vi "getConfiguration.vi"(8 "error in (no error)":errorcluster, 11 "Camera in":refnum<class "Camera.lvclass">) -> (0 "error out":errorcluster, 2 "configuration":T2={"exposure_time_s"=nan, "delay_time_s"=nan, "roi"={"x0"=18446744073709551615, "y0"=18446744073709551615, "x1"=18446744073709551615, "y1"=18446744073709551615}, "timestamp_mode"=65535, "pixelrate"=4294967295, "trigger_mode"=65535, "acquire_mode"=65535, "metadata_mode"=65535, "noisefilter_mode"=65535, "binning"={"vert"=65535, "horz"=65535}} {"noisefilter_mode" items=["Undefined"=65535, "OFF"=0, "ON"=1]; "exposure_time_s" format="%#_6f"; "timestamp_mode" items=["Undefined"=65535, "OFF"=0, "Binary"=1, "Binary+ASCII"=2, "ASCII"=3]; "acquire_mode" items=["Undefined"=65535, "auto"=0, "external"=1, "external modulate"=2]; "trigger_mode" items=["Undefined"=65535, "auto sequence"=0, "software trigger"=1, "external exposure start & software trigger"=2, "external exposure control"=3, "external synchronized"=4, "fast external exposure control"=5, "external CDS control"=6, "slow external exposure control"=7, "external synchronized HDSDI"=258]; "metadata_mode" items=["Undefined"=65535, "OFF"=0, "ON"=1]}, 3 "Camera out":refnum<class "Camera.lvclass">)   [LabVIEW 2019, in "Camera.lvclass"]
doc: "Gets the current configuration from the camera."
uses:
  Camera.lvclass
  pco.sdk/TimingControl/TimingControl.lvlib
  pco.sdk/ImageSensor/ImageSensor.lvlib
  pco.sdk/RecordingControl/RecordingControl.lvlib
  Controls/binning.ctl
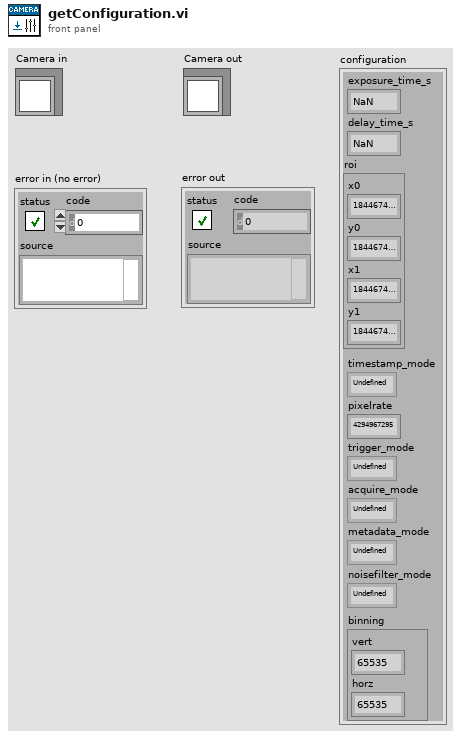
[diagram p1: front panel]
types:
  T1 = typedef "Camera.lvclass/binning.ctl" = cluster{"vert":u16, "horz":u16}
  T2 = cluster{"exposure_time_s":dbl, "delay_time_s":dbl, "roi":cluster{"x0":u64, "y0":u64, "x1":u64, "y1":u64}, "timestamp_mode":u16, "pixelrate":u32, "trigger_mode":u16, "acquire_mode":u16, "metadata_mode":u16, "noisefilter_mode":u16, "binning":T1}
  T3 = cluster{"exposure_time_s":dbl, "delay_time_s":dbl, "roi":cluster{"x0":u64, "y0":u64, "x1":u64, "y1":u64}, "timestamp_mode":u16, "pixelrate":u32, "trigger_mode":u16, "acquire_mode":u16, "metadata_mode":u16, "noisefilter_mode":u16, "binning":cluster{"vert":u16, "horz":u16}}
  T4 = cluster{"wSensorTypeDESC":u16, "wSensorSubTypeDESC":u16, "wMaxHorzResStdDESC":u16, "wMaxVertResStdDESC":u16, "wMaxHorzResExtDESC":u16, "wMaxVertResExtDESC":u16, "wDynResDESC":u16, "wMaxBinHorzDESC":u16, "wBinHorzSteppingDESC":u16, "wMaxBinVertDESC":u16, "wBinVertSteppingDESC":u16, "wRoiHorStepsDESC":u16, "wRoiVertStepsDESC":u16, "wNumADCsDESC":u16, "wMinSizeHorzDESC":u16, "dwPixelRateDESC":u32[], "wConvFactDESC":u16[], "sCoolingSetpoints":i16[], "wSoftRoiHorStepsDESC":u16, "wSoftRoiVertStepsDESC":u16, "wIRDESC":u16, "wMinSizeVertDESC":u16, "dwMinDelayDESC":u32, "dwMaxDelayDESC":u32, "dwMinDelayStepDESC":u32, "dwMinExposureDESC":u32, "dwMaxExposureDESC":u32, "dwMinExposureStepDESC":u32, "dwMinDelayIRDESC":u32, "dwMaxDelayIRDESC":u32, "dwMinExposureIRDESC":u32, "dwMaxExposureIRDESC":u32, "wTimeTableDESC":u16, "wDoubleImageDESC":u16, "sMinCoolSetDESC":i16, "sMaxCoolSetDESC":i16, "sDefaultCoolSetDESC":i16, "wPowerDownModeDESC":u16, "wOffsetRegulationDESC":u16, "wColorPatternDESC":u16, "wPatternTypeDESC":u16, "wNumCoolingSetpoints":u16, "dwGeneralCapsDESC1":u32, "dwGeneralCapsDESC2":u32, "dwExtSyncFrequency":u32[], "dwGeneralCapsDESC3":u32, "dwGeneralCapsDESC4":u32}
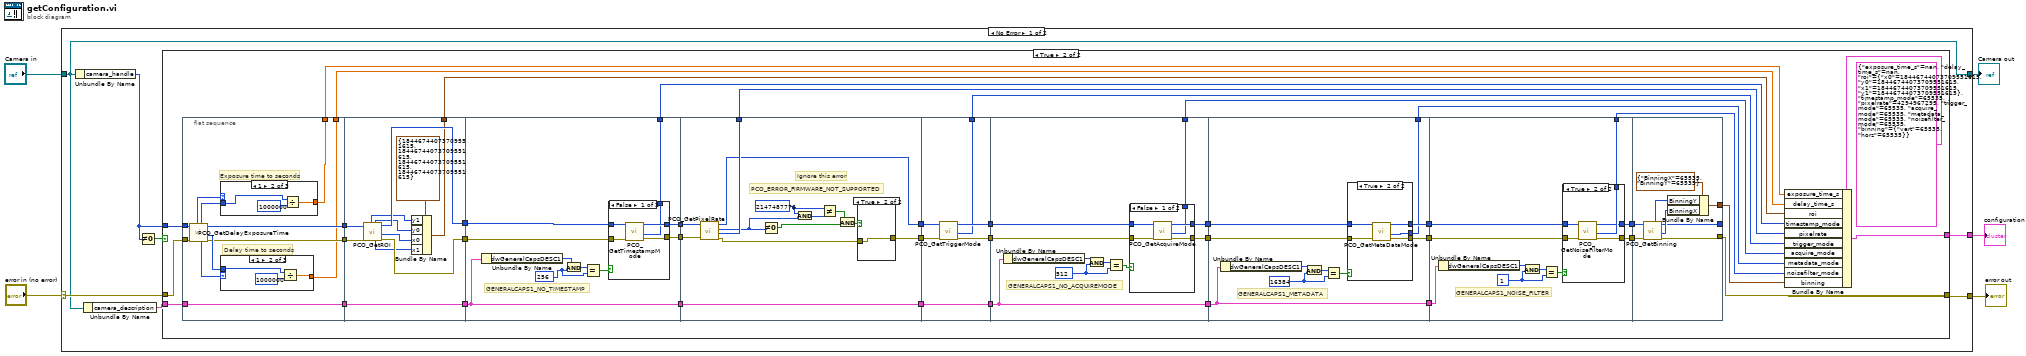
[diagram p0: block diagram]
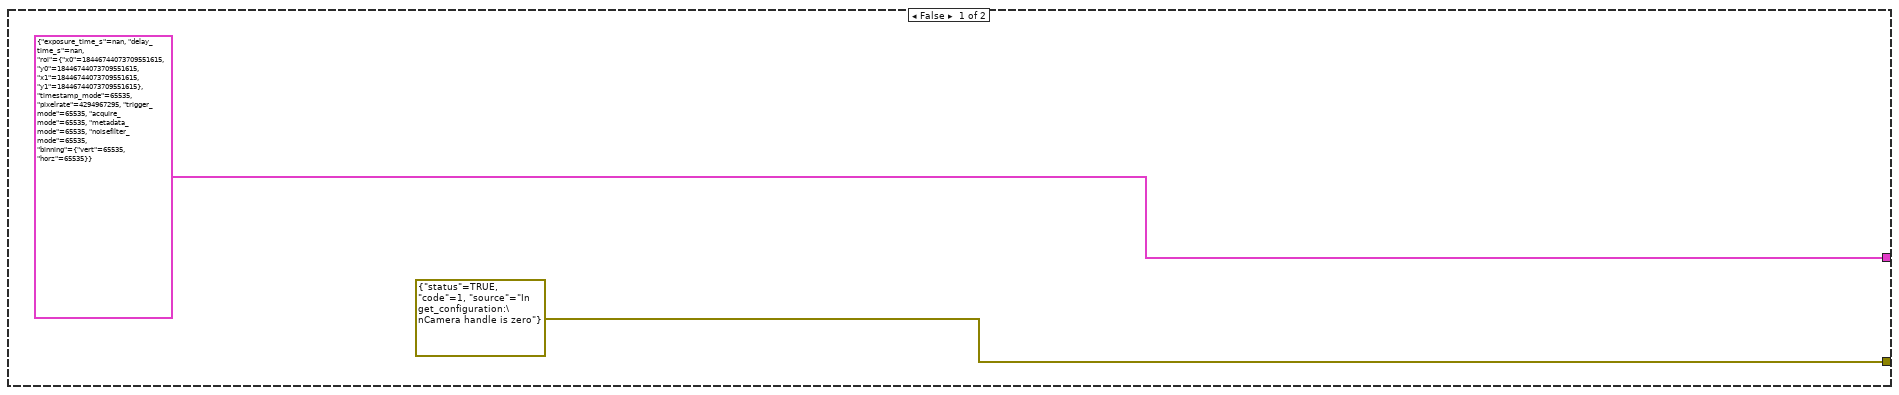
[diagram p2: hidden frame]
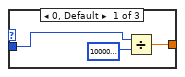
[diagram p3: hidden frame]
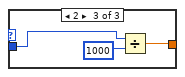
[diagram p4: hidden frame]
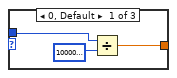
[diagram p5: hidden frame]
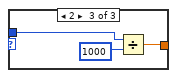
[diagram p6: hidden frame]
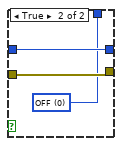
[diagram p7: hidden frame]
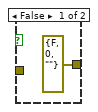
[diagram p8: hidden frame]
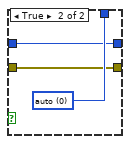
[diagram p9: hidden frame]
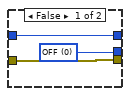
[diagram p10: hidden frame]
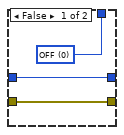
[diagram p11: hidden frame]
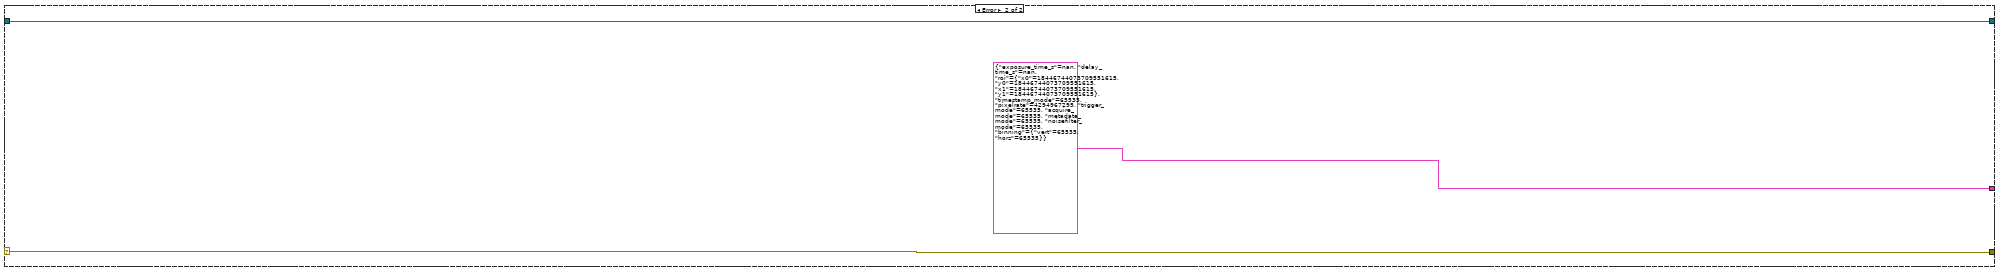
[diagram p12: hidden frame]
diagram:
  n1 = case shown="No Error" "error in (no error)" {
    selector: "error in (no error)" -> [w9 w197]
    tunnel: [w11 w197] -> w4
    tunnel: [w7 w196] -> w2
    tunnel: "Camera in" -> [w7 w196]
    tunnel: [w8 T3 {"exposure_time_s"=nan, "delay_time_s"=nan, "roi"={"x0"=18446744073709551615, "y0"=18446744073709551615, "x1"=18446744073709551615, "y1"=18446744073709551615}, "timestamp_mode"=65535, "pixelrate"=4294967295, "trigger_mode"=65535, "acquire_mode"=65535, "metadata_mode"=65535, "noisefilter_mode"=65535, "binning"={"vert"=65535, "horz"=65535}} ("configuration")] -> w1
    frame No Error {
      n2 = Unbundle By Name(w7) -> ("camera_handle"=w10:u64)
      n3 = Unbundle By Name(w7) -> ("camera_description"=w6:T4)
      n4 = Not Equal To 0?(x=w10) -> (x != 0?=w12:bool)
      n5 = case shown="True" w12 {
        tunnel: [errorcluster {"status"=TRUE, "code"=1, "source"="In get_configuration:\nCamera handle is zero"} ("error constant") w15] -> w11
        tunnel: w10 -> [_ w21]
        tunnel: w9 -> [_ w22]
        tunnel: [T3 {"exposure_time_s"=nan, "delay_time_s"=nan, "roi"={"x0"=18446744073709551615, "y0"=18446744073709551615, "x1"=18446744073709551615, "y1"=18446744073709551615}, "timestamp_mode"=65535, "pixelrate"=4294967295, "trigger_mode"=65535, "acquire_mode"=65535, "metadata_mode"=65535, "noisefilter_mode"=65535, "binning"={"vert"=65535, "horz"=65535}} ("configuration") w17] -> w8
        tunnel: w6 -> [_ w20]
        frame False {
        }
        frame True {
          n6 = flat-sequence {
            tunnel: [w60] -> w53
            tunnel: [w59] -> w52
            tunnel: [w58] -> w41
            tunnel: [w57] -> w40
            tunnel: [w54] -> w34
            tunnel: w22 -> [w56]
            tunnel: w21 -> [w55]
            tunnel: w20 -> [w54]
            tunnel: w53 -> [w92]
            tunnel: w52 -> [w93]
            tunnel: [w90] -> w51
            tunnel: [w89] -> w50
            tunnel: [w83] -> w19
            tunnel: [w84] -> w35
            tunnel: w34 -> [w84]
            tunnel: w51 -> [w102]
            tunnel: w50 -> [w103]
            tunnel: [w101] -> w49
            tunnel: [w100] -> w48
            tunnel: [w99] -> w39
            tunnel: w35 -> [w94]
            tunnel: [w94] -> w30
            tunnel: w49 -> [w124]
            tunnel: w48 -> [w123]
            tunnel: [w113] -> w45
            tunnel: [w112] -> w43
            tunnel: [w122] -> w38
            tunnel: [w121] -> w31
            tunnel: w30 -> [w121]
            tunnel: w45 -> [w132]
            tunnel: [w129] -> w44
            tunnel: w43 -> [w131]
            tunnel: [w130] -> w42
            tunnel: [w128] -> w37
            tunnel: [w127] -> w32
            tunnel: w31 -> [w127]
            tunnel: w44 -> [w142]
            tunnel: w42 -> [w141]
            tunnel: [w138] -> w36
            tunnel: [w140] -> w47
            tunnel: [w139] -> w46
            tunnel: [w134] -> w33
            tunnel: w32 -> [w134]
            tunnel: w47 -> [w153]
            tunnel: w46 -> [w152]
            tunnel: [w156] -> w28
            tunnel: [w155] -> w26
            tunnel: [w154] -> w29
            tunnel: w33 -> [w151]
            tunnel: [w151] -> w24
            tunnel: w28 -> [w172]
            tunnel: [w170] -> w27
            tunnel: w26 -> [w173]
            tunnel: [w169] -> w25
            tunnel: w24 -> [w175]
            tunnel: [w171] -> w23
            tunnel: w27 -> [w194]
            tunnel: w25 -> [w193]
            tunnel: [w189] -> _
            tunnel: [w188] -> w16
            tunnel: [w187] -> w15
            frame #0 {
              # "Delay time to seconds"
              # "Exposure time to seconds"
              n7 = call "PCO_GetDelayExposureTime.vi"("error in (no error)"=w56, "ph"=w55) -> ("error out"=w59:errorcluster, "dwDelay"=w61:u32, "ph out"=w60:u64, "wTimeBaseDelay"=w64:u16, "dwExposure"=w62:u32, "wTimeBaseExposure"=w63:u16)  [unwired: 3 in, 1 out]
              n8 = case shown="1" w63 {
                tunnel: w62 -> [w66 w69 w72]
                tunnel: [w65 w68 w71] -> w58
                frame 0, Default {
                  n9 = Divide(x=w66, y=u32 1000000000) -> (x/y=w65:dbl)
                }
                frame 1 {
                  n10 = Divide(x=w69, y=u32 1000000) -> (x/y=w68:dbl)
                }
                frame 2 {
                  n11 = Divide(x=w72, y=u32 1000) -> (x/y=w71:dbl)
                }
              }
              n12 = case shown="1" w64 {
                tunnel: w61 -> [w76 w78 w81]
                tunnel: [w74 w77 w80] -> w57
                frame 0, Default {
                  n13 = Divide(x=w76, y=u32 1000000000) -> (x/y=w74:dbl)
                }
                frame 1 {
                  n14 = Divide(x=w78, y=u32 1000000) -> (x/y=w77:dbl)
                }
                frame 2 {
                  n15 = Divide(x=w81, y=u32 1000) -> (x/y=w80:dbl)
                }
              }
            }
            frame #1 {
              n16 = call "PCO_GetROI.vi"("error in (no error)"=w93, "ph"=w92) -> ("error out"=w90:errorcluster, "wRoiX0"=w88:u16, "ph out"=w89:u64, "wRoiX1"=w87:u16, "wRoiY0"=w86:u16, "wRoiY1"=w85:u16)  [unwired: 3 in, 1 out]
              n17 = Bundle By Name(cluster=cluster{"x0":u64, "y0":u64, "x1":u64, "y1":u64} {"x0"=18446744073709551615, "y0"=18446744073709551615, "x1"=18446744073709551615, "y1"=18446744073709551615}, "y1"=w85, "y0"=w86, "x0"=w88, "x1"=w87) -> (w83:cluster{"x0":u64, "y0":u64, "x1":u64, "y1":u64})
            }
            frame #2 {
              w96 = u32 256 ("y")
              # "GENERALCAPS1_NO_TIMESTAMP"
              n18 = Unbundle By Name(w94) -> ("dwGeneralCapsDESC1"=w97:u32)
              n19 = And(x=w97, y=w96) -> (x .and. y?=w98:u32)
              n20 = Equal?(x=w98, y=w96) -> (x = y?=w95:bool)
              n21 = case shown="False" w95 {
                tunnel: w103 -> [w108 w111]
                tunnel: w102 -> [w107 w110]
                tunnel: [w106 w110] -> w101
                tunnel: [w105 w111] -> w100
                tunnel: [w104 w109] -> w99
                frame False {
                  n22 = call "PCO_GetTimestampMode.vi"("error in (no error)"=w107, "ph"=w108) -> ("error out"=w106:errorcluster, "wTimeStampMode"=w104:u16, "ph out"=w105:u64)  [unwired: 6 in, 1 out]
                }
                frame True {
                  w109 = u16 0 items=["OFF", "Binary", "Binary+ASCII", "ASCII"] ("wTimeStampMode")
                }
              }
            }
            frame #3 {
              w118 = u32 2147487776
              # "Ignore this error"
              # "PCO_ERROR_FIRMWARE_NOT_SUPPORTED"
              n23 = call "PCO_GetPixelRate.vi"("error in (no error)"=w124, "ph"=w123) -> ("error out"=w114:errorcluster, "dwPixelRate"=w122:u32, "ErrorMessage"=w120:i32, "ph out"=w112:u64)  [unwired: 6 in]
              n24 = Not Equal To 0?(x=w120) -> (x != 0?=w116:bool)
              n25 = And(x=w118, y=w120) -> (x .and. y?=w119:u32)
              n26 = Not Equal?(x=w118, y=w119) -> (x != y?=w117:bool)
              n27 = And(x=w117, y=w116) -> (x .and. y?=w115:bool)
              n28 = case shown="True" w115 {
                tunnel: w114 -> [_ w126]
                tunnel: [errorcluster {"status"=FALSE, "code"=0, "source"=""} ("error out") w126] -> w113
                frame False {
                }
                frame True {
                }
              }
            }
            frame #4 {
              n29 = call "PCO_GetTriggerMode.vi"("error in (no error)"=w132, "ph"=w131) -> ("error out"=w129:errorcluster, "wTriggerMode"=w128:u16, "ph out"=w130:u64)  [unwired: 6 in, 1 out]
            }
            frame #5 {
              w135 = u32 512 ("y")
              # "GENERALCAPS1_NO_ACQUIREMODE"
              n30 = Unbundle By Name(w134) -> ("dwGeneralCapsDESC1"=w137:u32)
              n31 = And(x=w137, y=w135) -> (x .and. y?=w136:u32)
              n32 = Equal?(x=w136, y=w135) -> (x = y?=w133:bool)
              n33 = case shown="False" w133 {
                tunnel: w142 -> [w147 w148]
                tunnel: w141 -> [w146 w149]
                tunnel: [w145 w149] -> w140
                tunnel: [w144 w148] -> w139
                tunnel: [w143 w150] -> w138
                frame False {
                  n34 = call "PCO_GetAcquireMode.vi"("error in (no error)"=w147, "ph"=w146) -> ("error out"=w144:errorcluster, "wAcquMode"=w143:u16, "ph out"=w145:u64)  [unwired: 6 in, 1 out]
                }
                frame True {
                  w150 = u16 0 items=["auto", "external", "external modulate"] ("wAcquMode")
                }
              }
            }
            frame #6 {
              w158 = u32 16384 ("y")
              # "GENERALCAPS1_METADATA"
              n35 = Unbundle By Name(w151) -> ("dwGeneralCapsDESC1"=w160:u32)
              n36 = And(x=w160, y=w158) -> (x .and. y?=w159:u32)
              n37 = Equal?(x=w159, y=w158) -> (x = y?=w157:bool)
              n38 = case shown="True" w157 {
                tunnel: w153 -> [w163 w168]
                tunnel: w152 -> [w161 w167]
                tunnel: [w163 w166] -> w156
                tunnel: [w161 w165] -> w155
                tunnel: [w162 w164] -> w154
                frame False {
                  w162 = u16 0 items=["OFF", "ON"] ("wMetaDataMode")
                }
                frame True {
                  n39 = call "PCO_GetMetaDataMode.vi"("error in (no error)"=w167, "ph"=w168) -> ("error out"=w165:errorcluster, "wMetaDataMode"=w164:u16, "ph out"=w166:u64)  [unwired: 4 in, 3 out]
                }
              }
            }
            frame #7 {
              w176 = u32 1 ("y")
              # "GENERALCAPS1_NOISE_FILTER"
              n40 = Unbundle By Name(w175) -> ("dwGeneralCapsDESC1"=w178:u32)
              n41 = And(x=w178, y=w176) -> (x .and. y?=w177:u32)
              n42 = Equal?(x=w177, y=w176) -> (x = y?=w174:bool)
              n43 = case shown="True" w174 {
                tunnel: w173 -> [w179 w186]
                tunnel: w172 -> [w180 w185]
                tunnel: [w181 w184] -> w171
                tunnel: [w180 w183] -> w170
                tunnel: [w179 w182] -> w169
                frame False {
                  w181 = u16 0 items=["OFF", "ON"] ("noisefilter_mode")
                }
                frame True {
                  n44 = call "PCO_GetNoiseFilterMode.vi"("error in (no error)"=w186, "ph"=w185) -> ("error out"=w182:errorcluster, "wNoiseFilterMode"=w184:u16, "ph out"=w183:u64)  [unwired: 6 in, 1 out]
                }
              }
            }
            frame #8 {
              n45 = call "PCO_GetBinning.vi"("error in (no error)"=w193, "ph"=w194) -> ("error out"=w187:errorcluster, "wBinHorz"=w190:u16, "ph out"=w189:u64, "wBinVert"=w191:u16)  [unwired: 5 in, 1 out]
              n46 = Bundle By Name(cluster=cluster{"BinningX":u16, "BinningY":u16} {"BinningX"=65535, "BinningY"=65535} ("Binning"), "BinningY"=w191, "BinningX"=w190) -> (w188:cluster{"BinningX":u16, "BinningY":u16})
            }
          }
          n47 = Bundle By Name(cluster=T3 {"exposure_time_s"=nan, "delay_time_s"=nan, "roi"={"x0"=18446744073709551615, "y0"=18446744073709551615, "x1"=18446744073709551615, "y1"=18446744073709551615}, "timestamp_mode"=65535, "pixelrate"=4294967295, "trigger_mode"=65535, "acquire_mode"=65535, "metadata_mode"=65535, "noisefilter_mode"=65535, "binning"={"vert"=65535, "horz"=65535}} ("configuration"), "exposure_time_s"=w41, "delay_time_s"=w40, "roi"=w19, "timestamp_mode"=w39, "pixelrate"=w38, "trigger_mode"=w37, "acquire_mode"=w36, "metadata_mode"=w29, "noisefilter_mode"=w23, "binning"=w16) -> (w17:T3)
        }
      }
    }
    frame Error {
    }
  }
  "error out" <- w4
  "Camera out" <- w2
  "configuration" <- w1
